vi "Digital Output.vi"(4 "Check Byte/Word (F:Byte)":bool, 6 "Check Digital Port (F:Port 1)":bool, 7 "Slot Number (1)":u8=1 min=1 max=3 step=1, 8 "error in (no error)":errorcluster, 9 "DIO Write (All F:0)":bool[](array[boolean]), 10 "Set/Check (F:Set)":bool, 11 "VISA Resource Name":refnum<visa-resource-name>) -> (0 "error out":errorcluster, 2 "DIO Check":bool[](array[boolean]), 3 "VISA Resource Name Out":refnum<visa-resource-name>)   [LabVIEW 2012, in "Agilent 34970.lvlib"]
doc: "This VI allows you to set or check the output of digital ports on the HP34970A Multifunction module."
uses:
  <instrlib>/Agilent 34970/Agilent 34970.lvlib
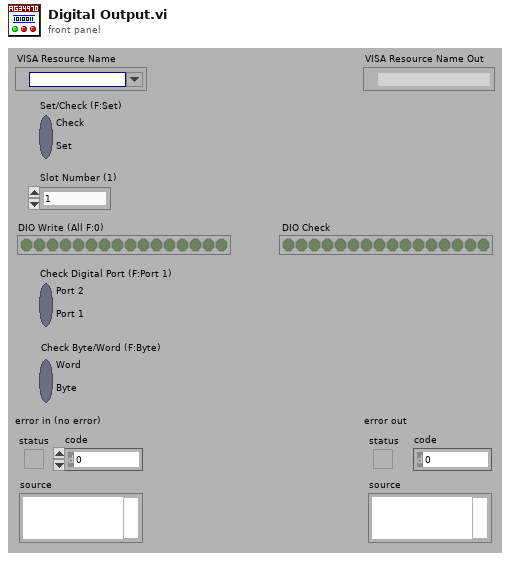
[diagram p1: front panel]
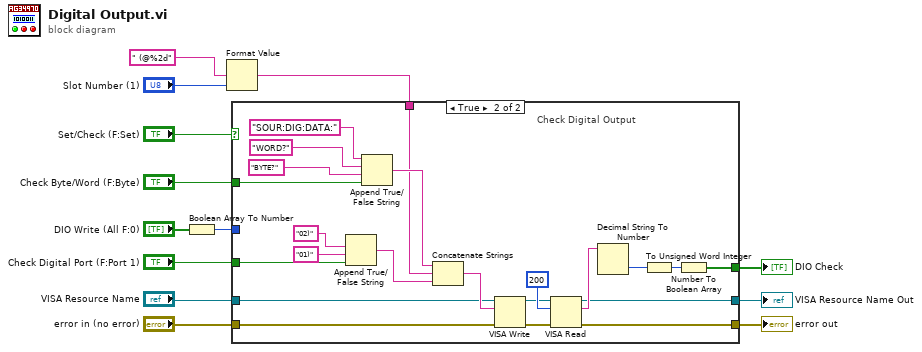
[diagram p0: block diagram]
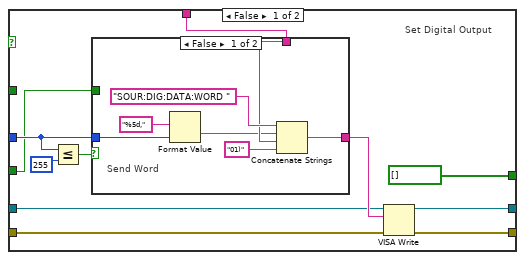
[diagram p2: hidden frame]
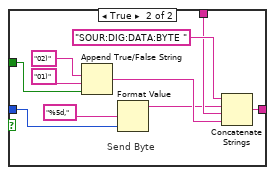
[diagram p3: hidden frame]
diagram:
  n1 = Boolean Array To Number(Boolean array="DIO Write (All F:0)") -> (number=w8:u32)
  n2 = Format Value(format string=" (@%2d", value (0)="Slot Number (1)") -> (output string=w9:string)  [unwired: 1 in]
  n3 = case shown="True" "Set/Check (F:Set)" {
    tunnel: [bool[] [] ("Boolean array") w42] -> w2
    tunnel: w9 -> [w23 w51]
    tunnel: w8 -> [w22 _]
    tunnel: "VISA Resource Name" -> [w20 w44]
    tunnel: "error in (no error)" -> [w19 w43]
    tunnel: [w18 w46] -> w3
    tunnel: [w17 w45] -> w4
    tunnel: "Check Byte/Word (F:Byte)" -> [_ w56]
    tunnel: "Check Digital Port (F:Port 1)" -> [w14 w54]
    frame False {
      # "Set Digital Output"
      n4 = Less Or Equal?(x=w22, y=u32 255) -> (x <= y?=w24:bool)
      n5 = case shown="False" w24 {
        tunnel: w22 -> [w28 w36]
        tunnel: [w27 w35] -> w21
        tunnel: w23 -> [w26 w33]
        tunnel: w14 -> [_ w34]
        frame False {
          # "Send Word"
          n6 = Format Value(format string="%5d,", value (0)=w28) -> (output string=w25:string)  [unwired: 1 in]
          n7 = Concatenate Strings("SOUR:DIG:DATA:WORD ", w25, w26, "01)") -> (w27:string)
        }
        frame True {
          # "Send Byte"
          n8 = Append True/False String(1:w34, 2:"01)" ("false string"), 3:"02)" ("true string")) -> (0:w38:string)  [unwired: 1 in]
          n9 = Format Value(format string="%5d,", value (0)=w36) -> (output string=w32:string)  [unwired: 1 in]
          n10 = Concatenate Strings("SOUR:DIG:DATA:BYTE ", w32, w33, w38) -> (w35:string)
        }
      }
      n11 = VISA Write(VISA resource name=w20, write buffer=w21, error in (no error)=w19) -> (VISA resource name out=w18:refnum<visa-resource-name>, error out=w17:errorcluster)  [unwired: 1 out]
    }
    frame True {
      # "Check Digital Output"
      n12 = Append True/False String(1:w54, 2:"01)" ("false string"), 3:"02)" ("false string")) -> (0:w48:string)  [unwired: 1 in]
      n13 = Append True/False String(1:w56, 2:"BYTE?" ("false string"), 3:"WORD?" ("true string"), 4:"SOUR:DIG:DATA:") -> (0:w52:string)
      n14 = Concatenate Strings(w52, w51, w48) -> (w53:string)
      n15 = VISA Write(VISA resource name=w44, write buffer=w53, error in (no error)=w43) -> (VISA resource name out=w62:refnum<visa-resource-name>, error out=w61:errorcluster)  [unwired: 1 out]
      n16 = VISA Read(VISA resource name=w62, byte count=u32 200 ("byte count (0)"), error in (no error)=w61) -> (VISA resource name out=w46:refnum<visa-resource-name>, read buffer=w47:string, error out=w45:errorcluster)  [unwired: 1 out]
      n17 = Decimal String To Number(string=w47) -> (number=w59:i32)  [unwired: 2 in, 1 out]
      n18 = To Unsigned Word Integer(number=w59) -> (unsigned 16bit integer=w60:u16)
      n19 = Number To Boolean Array(number=w60) -> (Boolean array=w42:bool[])
    }
  }
  "DIO Check" <- w2
  "error out" <- w4
  "VISA Resource Name Out" <- w3
